vi "Write Datalog To File.vi"(0 "State":string, 1 "Datalog?":bool, 2 "File Ref":refnum<file>, 5 "Quantity":i32, 7 "Ingredient":string, 9 "Beverage Name":string, 11 "Error In":errorcluster) -> (4 "Datalog String":string, 15 "Error Out":errorcluster)   [LabVIEW 2020]
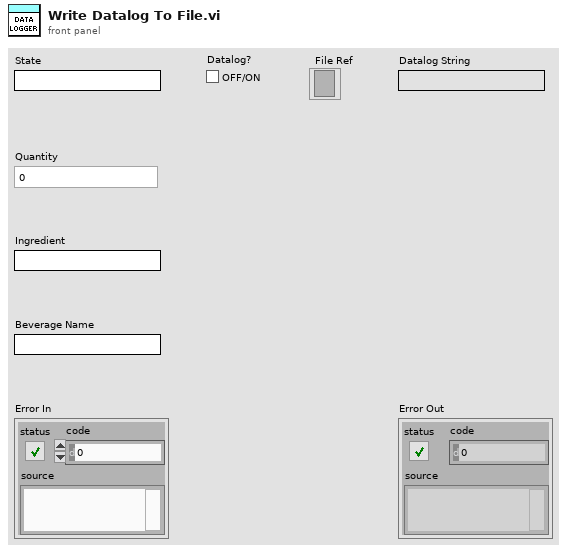
[diagram p1: front panel]
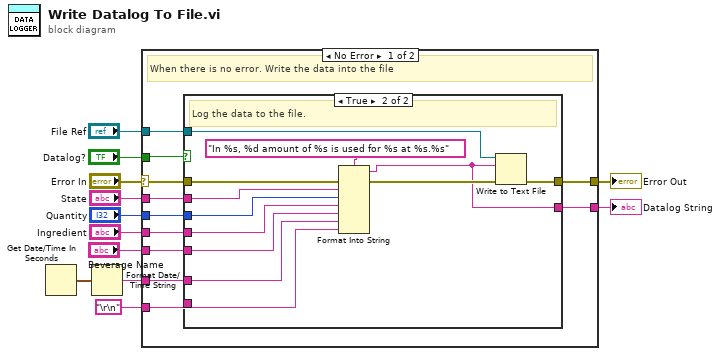
[diagram p0: block diagram]
diagram:
  n1 = Get Date/Time In Seconds() -> (seconds since 1Jan1904=w5:timestamp)
  n2 = Format Date/Time String(seconds (now)=w5) -> (date/time string=w4:string)  [unwired: 2 in]
  n3 = case shown="No Error" "Error In" {
    selector: "Error In" -> [w20 w37]
    tunnel: [w19 w37] -> w11
    tunnel: "State" -> [w23 _]
    tunnel: "Quantity" -> [w22 _]
    tunnel: "Ingredient" -> [w21 _]
    tunnel: "\r\n" -> [w17 _]
    tunnel: "File Ref" -> [w18 _]
    tunnel: w4 -> [w16 _]
    tunnel: "Datalog?" -> [w15 _]
    tunnel: [w14 _] -> w2
    tunnel: "Beverage Name" -> [w13 _]
    frame No Error {
      # "When there is no error. Write the data into the file"
      n4 = case shown="True" w15 {
        tunnel: w23 -> [_ w34]
        tunnel: w22 -> [_ w33]
        tunnel: w21 -> [_ w32]
        tunnel: w20 -> [w24 w31]
        tunnel: [w24 w30] -> w19
        tunnel: w18 -> [_ w29]
        tunnel: w17 -> [_ w28]
        tunnel: w16 -> [_ w26]
        tunnel: [_ w27] -> w14
        tunnel: w13 -> [_ w25]
        frame False {
          # "Don't log the data into the file"
        }
        frame True {
          # "Log the data to the file."
          n5 = Format Into String(format string="In %s, %d amount of %s is used for %s at %s.%s", error in=w31, w34, w33, w32, w25, w26, w28) -> (resulting string=w27:string, error out=w36:errorcluster)  [unwired: 1 in]
          n6 = Write to Text File(file (use dialog)=w29, text=w27, error in=w36) -> (error out=w30:errorcluster)  [unwired: 1 in, 2 out]
        }
      }
    }
    frame Error {
      # "When there is error. Do nothing"
    }
  }
  "Error Out" <- w11
  "Datalog String" <- w2
